vi "GenerateAndBoundKukaMotions.vi"(1 "Output Array":dbl[](array[numeric])=[200.0, -350.0, 128.0, -180.0, 0.0, 90.0]) -> (0 "Output Array":dbl[](array[numeric]))   [LabVIEW 2011]
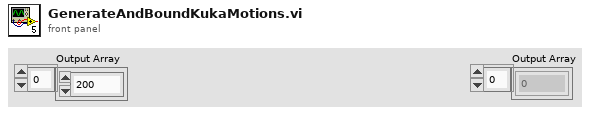
[diagram p1: front panel]
types:
  T1 = enum16{"Position & Angles", "Angles", "Position"}
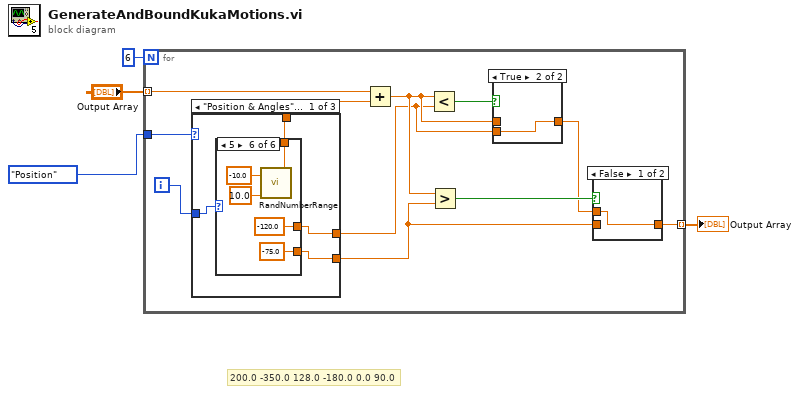
[diagram p0: block diagram]
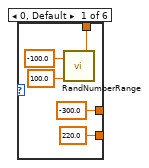
[diagram p2: hidden frame]
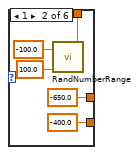
[diagram p3: hidden frame]
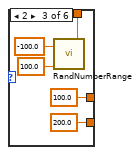
[diagram p4: hidden frame]
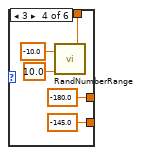
[diagram p5: hidden frame]
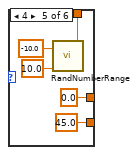
[diagram p6: hidden frame]
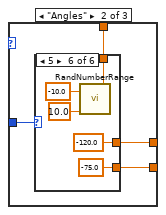
[diagram p7: hidden frame]
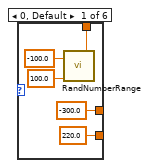
[diagram p8: hidden frame]
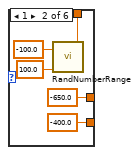
[diagram p9: hidden frame]
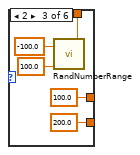
[diagram p10: hidden frame]
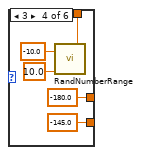
[diagram p11: hidden frame]
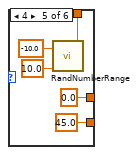
[diagram p12: hidden frame]
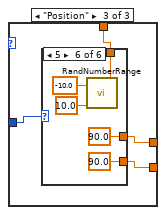
[diagram p13: hidden frame]
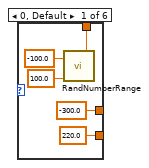
[diagram p14: hidden frame]
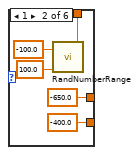
[diagram p15: hidden frame]
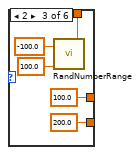
[diagram p16: hidden frame]
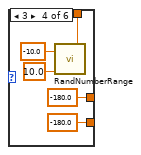
[diagram p17: hidden frame]
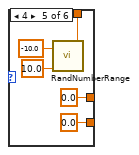
[diagram p18: hidden frame]
diagram:
  # "200.0 -350.0 128.0 -180.0 0.0 90.0"
  n1 = for {
    N: 6 -> [_]
    tunnel: "Output Array" -> [w14] mode=indexing
    tunnel: [w7] -> w2 mode=indexing
    tunnel: T1."Position" -> [w5]
    i -> [w15]
    n2 = case shown="\"Position & Angles\", Default" w5 {
      tunnel: w15 -> [w16 w53 w84]
      tunnel: [w18 w52 w86] -> w10
      tunnel: [w17 w51 w85] -> w8
      tunnel: [w19 w50 w87] -> w6
      frame "Position & Angles", Default {
        n3 = case shown="5" w16 {
          tunnel: [-300.0 ("Min") -650.0 ("Min") 100.0 ("Min") -180.0 ("Min") 0.0 ("Min") -120.0 ("Min")] -> w18
          tunnel: [220.0 ("Min") -400.0 ("Min") 200.0 ("Min") -145.0 ("Min") 45.0 ("Min") -75.0 ("Min")] -> w17
          tunnel: [w20 w25 w30 w35 w40 w45] -> w19
          frame 0, Default {
            n4 = call "RandNumberRange.vi"("Max"=100.0, "Min"=-100.0) -> ("Value"=w20:dbl)
          }
          frame 1 {
            n5 = call "RandNumberRange.vi"("Max"=100.0, "Min"=-100.0) -> ("Value"=w25:dbl)
          }
          frame 2 {
            n6 = call "RandNumberRange.vi"("Max"=100.0, "Min"=-100.0) -> ("Value"=w30:dbl)
          }
          frame 3 {
            n7 = call "RandNumberRange.vi"("Max"=10.0, "Min"=-10.0) -> ("Value"=w35:dbl)
          }
          frame 4 {
            n8 = call "RandNumberRange.vi"("Max"=10.0, "Min"=-10.0) -> ("Value"=w40:dbl)
          }
          frame 5 {
            n9 = call "RandNumberRange.vi"("Max"=10.0, "Min"=-10.0) -> ("Value"=w45:dbl)
          }
        }
      }
      frame "Angles" {
        n10 = case shown="5" w53 {
          tunnel: [-300.0 ("Min") -650.0 ("Min") 100.0 ("Min") -180.0 ("Min") 0.0 ("Min") -120.0 ("Min")] -> w52
          tunnel: [220.0 ("Min") -400.0 ("Min") 200.0 ("Min") -145.0 ("Min") 45.0 ("Min") -75.0 ("Min")] -> w51
          tunnel: [w54 w59 w64 w69 w74 w79] -> w50
          frame 0, Default {
            n11 = call "RandNumberRange.vi"("Max"=100.0, "Min"=-100.0) -> ("Value"=w54:dbl)
          }
          frame 1 {
            n12 = call "RandNumberRange.vi"("Max"=100.0, "Min"=-100.0) -> ("Value"=w59:dbl)
          }
          frame 2 {
            n13 = call "RandNumberRange.vi"("Max"=100.0, "Min"=-100.0) -> ("Value"=w64:dbl)
          }
          frame 3 {
            n14 = call "RandNumberRange.vi"("Max"=10.0, "Min"=-10.0) -> ("Value"=w69:dbl)
          }
          frame 4 {
            n15 = call "RandNumberRange.vi"("Max"=10.0, "Min"=-10.0) -> ("Value"=w74:dbl)
          }
          frame 5 {
            n16 = call "RandNumberRange.vi"("Max"=10.0, "Min"=-10.0) -> ("Value"=w79:dbl)
          }
        }
      }
      frame "Position" {
        n17 = case shown="5" w84 {
          tunnel: [-300.0 ("Min") -650.0 ("Min") 100.0 ("Min") -180.0 ("Min") 0.0 ("Min") 90.0 ("Min")] -> w86
          tunnel: [220.0 ("Min") -400.0 ("Min") 200.0 ("Min") -180.0 ("Min") 0.0 ("Min") 90.0 ("Min")] -> w85
          tunnel: [w88 w93 w98 w103 w108 w113] -> w87
          frame 0, Default {
            n18 = call "RandNumberRange.vi"("Max"=100.0, "Min"=-100.0) -> ("Value"=w88:dbl)
          }
          frame 1 {
            n19 = call "RandNumberRange.vi"("Max"=100.0, "Min"=-100.0) -> ("Value"=w93:dbl)
          }
          frame 2 {
            n20 = call "RandNumberRange.vi"("Max"=100.0, "Min"=-100.0) -> ("Value"=w98:dbl)
          }
          frame 3 {
            n21 = call "RandNumberRange.vi"("Max"=10.0, "Min"=-10.0) -> ("Value"=w103:dbl)
          }
          frame 4 {
            n22 = call "RandNumberRange.vi"("Max"=10.0, "Min"=-10.0) -> ("Value"=w108:dbl)
          }
          frame 5 {
            n23 = call "RandNumberRange.vi"("Max"=10.0, "Min"=-10.0) -> ("Value"=w113:dbl)
          }
        }
      }
    }
    n24 = Add(x=w14, y=w6) -> (x+y=w11:dbl)
    n25 = Less?(x=w11, y=w10) -> (x < y?=w13:bool)
    n26 = Greater?(x=w11, y=w8) -> (0:w12:bool)
    n27 = case shown="True" w13 {
      tunnel: [w120 w121] -> w9
      tunnel: w11 -> [w120 _]
      tunnel: w10 -> [_ w121]
      frame False {
      }
      frame True {
      }
    }
    n28 = case shown="False" w12 {
      tunnel: w9 -> [w118 _]
      tunnel: [w118 w119] -> w7
      tunnel: w8 -> [_ w119]
      frame False {
      }
      frame True {
      }
    }
  }
  "Output Array" <- w2
